vi "SDO_SIM_SIM_Execute.vi"(6 "FPGA_Time_Seconds":dbl, 8 "error in (no error)":errorcluster) -> (0 "error out":errorcluster)   [LabVIEW 2019]
uses:
  <vilib>/Rock Robotics/WPI/ThirdParty/JAS_Junk/TrajLib/VI/Util_GetTime_U32.vi
  <vilib>/Rock Robotics/WPI/ThirdParty/JAS_Junk/TrajLib/Conv_Radians_Deg.vi
  <vilib>/Rock Robotics/WPI/ThirdParty/JAS_Junk/TrajLib/BatterySim_CalculateLoadedBatteryVoltage.vi
  <vilib>/Rock Robotics/WPI/ThirdParty/JAS_Junk/TrajLib/VI/Util_GetTime_U64.vi
  Swerve_Drive_System/SDO_DRIVE_GLOBALS.vi
  SDO_SIM_SIM_Globals.vi
  <vilib>/Rock Robotics/WPI/ThirdParty/JAS_Junk/TrajLib/Trajectory_Library.lvlib
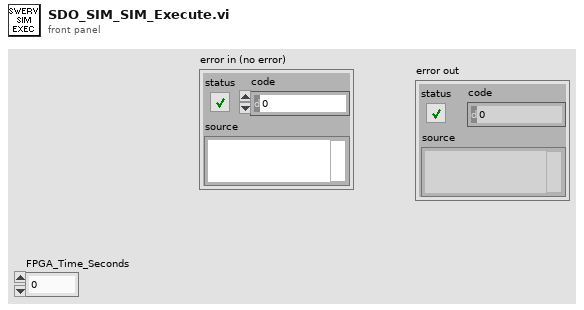
[diagram p1: front panel]
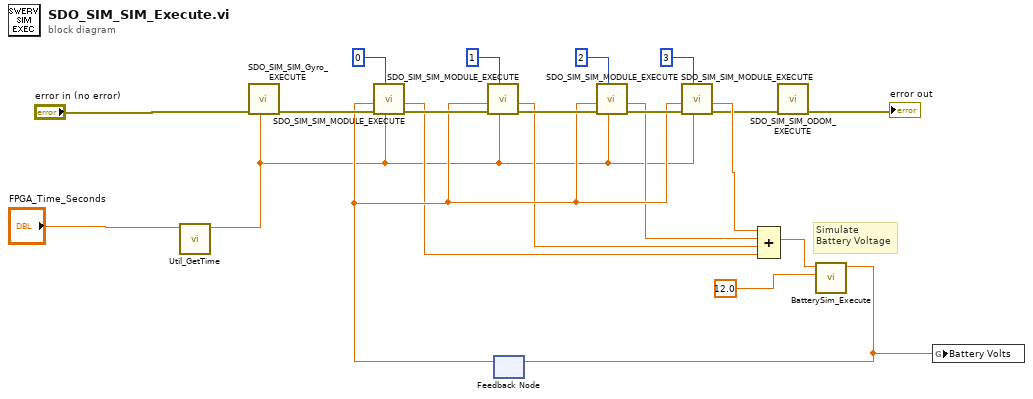
[diagram p0: block diagram]
diagram:
  # "Simulate\nBattery Voltage"
  n1 = call <vilib>:"Util_GetTime.vi"("Pass_Through_Time"="FPGA_Time_Seconds") -> ("FPGA_Time_Seconds"=w4:dbl)  [unwired: 8 in, 2 out]
  n2 = call "SDO_SIM_SIM_Gyro_EXECUTE.vi"("FPGA_Time_Seconds"=w4, "error in (no error)"="error in (no error)") -> ("error out"=w19:errorcluster)  [unwired: 9 in]
  n3 = feedback #1() -> (w8:dbl)  [unwired: 1 in]
  n4 = call "SDO_SIM_SIM_MODULE_EXECUTE.vi"("FPGA_Time_Seconds"=w4, "Module Index"=0, "error in (no error)"=w19, "Battery Voltage"=w8) -> ("error out"=w18:errorcluster, "Abs Current"=w5:dbl)  [unwired: 4 in, 2 out]
  n5 = call "SDO_SIM_SIM_MODULE_EXECUTE.vi"("FPGA_Time_Seconds"=w4, "Module Index"=1, "error in (no error)"=w18, "Battery Voltage"=w8) -> ("error out"=w17:errorcluster, "Abs Current"=w6:dbl)  [unwired: 4 in, 2 out]
  n6 = call "SDO_SIM_SIM_MODULE_EXECUTE.vi"("FPGA_Time_Seconds"=w4, "Module Index"=2, "error in (no error)"=w17, "Battery Voltage"=w8) -> ("error out"=w16:errorcluster, "Abs Current"=w7:dbl)  [unwired: 4 in, 2 out]
  n7 = call "SDO_SIM_SIM_MODULE_EXECUTE.vi"("FPGA_Time_Seconds"=w4, "Module Index"=3, "error in (no error)"=w16, "Battery Voltage"=w8) -> ("error out"=w2:errorcluster, "Abs Current"=w11:dbl)  [unwired: 4 in, 2 out]
  n8 = Compound Arithmetic op=ADD(w11, w7, w6, w5) -> (w10:dbl)
  n9 = call "SDO_SIM_SIM_ODOM_EXECUTE.vi"("error in (no error)"=w2) -> ("error out"=→"error out":errorcluster)  [unwired: 10 in]
  n10 = call <vilib>:"BatterySim_Execute.vi"("Nominal Battery Voltage"=12.0, "Current"=w10) -> ("Voltage"=w3:dbl)  [unwired: 9 in]
  n11 = feedback-in #1(w3) -> ()
  n12 = global write "SDO_SIM_SIM_Globals.vi" "Battery Volts"(w3) -> ()
